vi "Loop Till Force Sensed V2.vi"() -> ()   [LabVIEW 2013]
uses:
  <vilib>/Analysis/baseanly.llb/Mean (DBL).vi
  <vilib>/LabVIEW Interface for Arduino/LabVIEW Interface for Arduino.lvlib
  <vilib>/Analysis/NI_AALBase.lvlib
panel:
  out "Force Threshhold Reached":bool
  out "Force Average":dbl format="%0.2f"
  out "Force vs Time":dbl(graph)
  out "Voltage Average":dbl format="%0.2f"
  in  "Array":dbl[](array[numeric])
  in  "Analog Input Pin":u8
  in  "Stop":bool
  out "Volatege vs Time":dbl(graph)
  out "output array":dbl[](array[numeric])
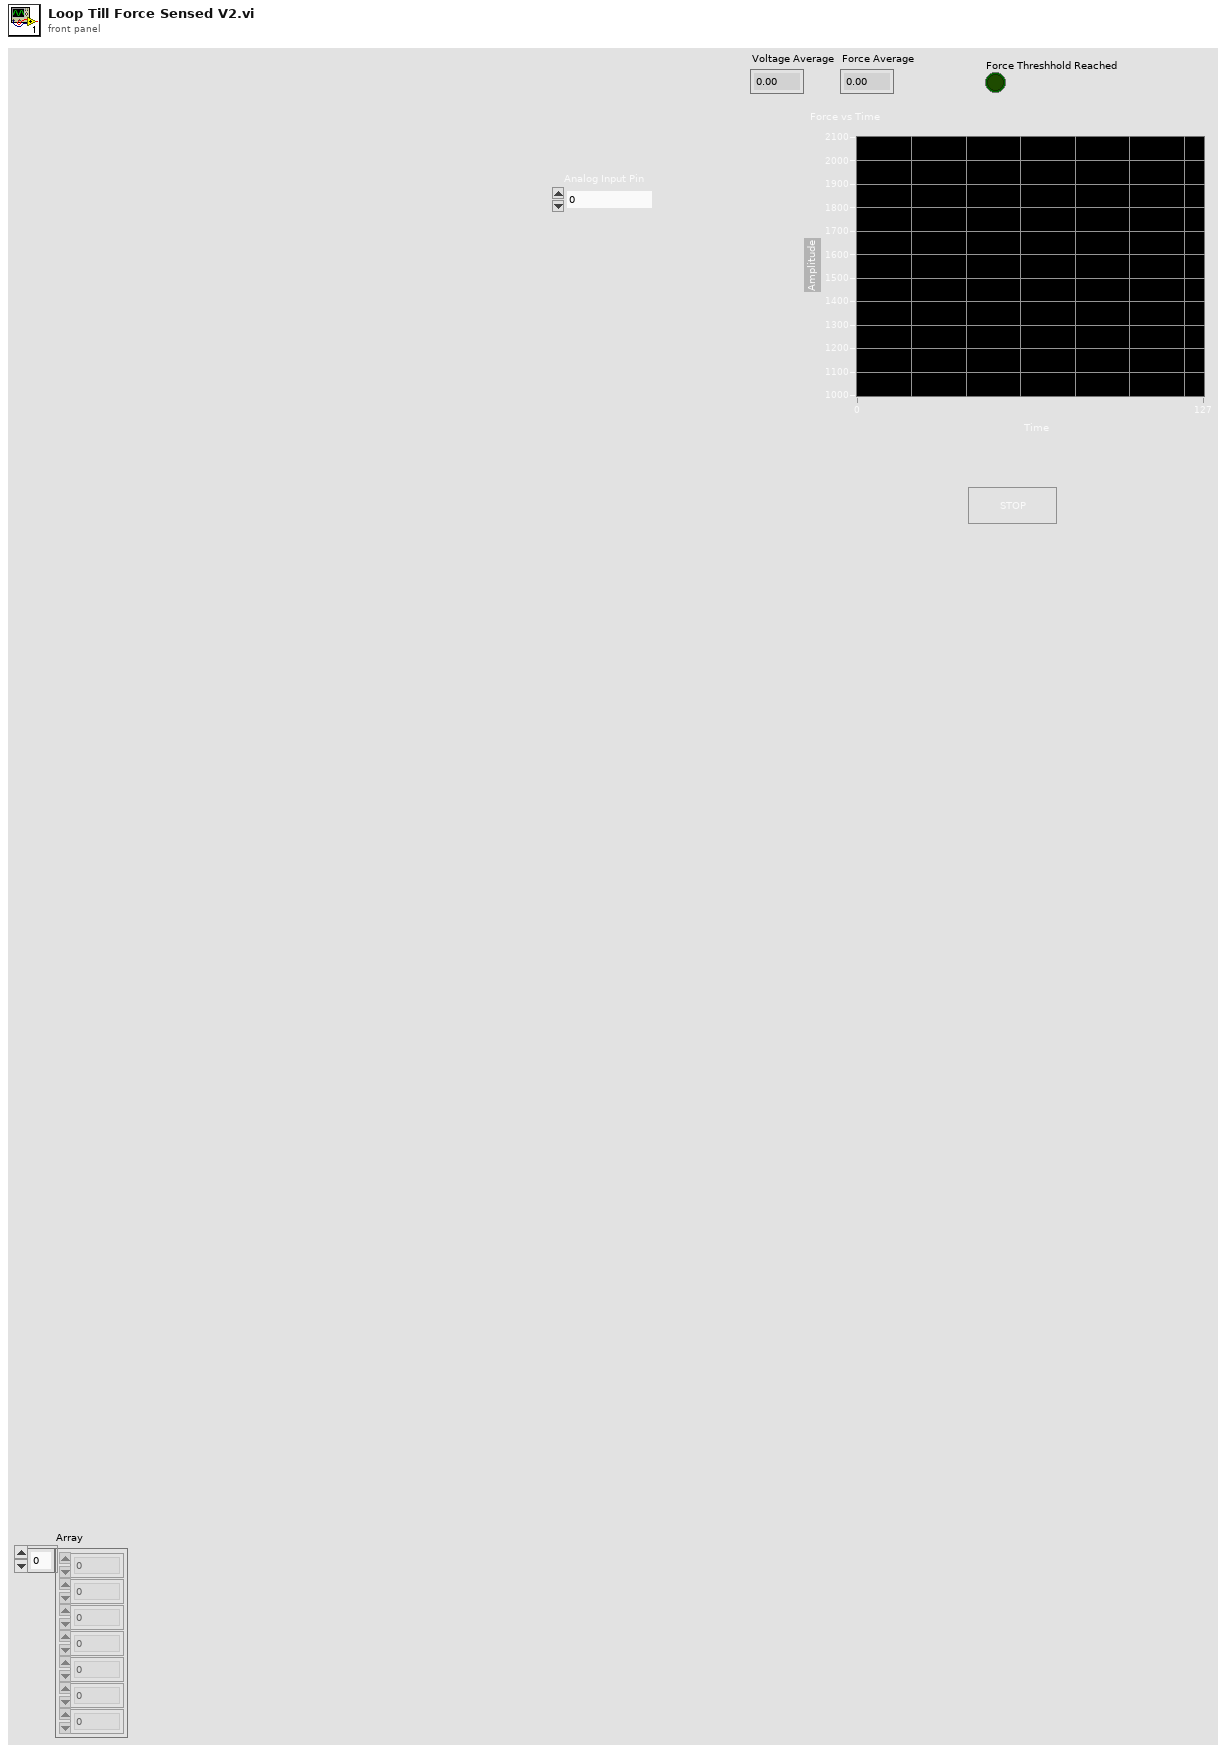
[diagram p1: front panel]
types:
  T1 = typedef "LabVIEW Interface for Arduino.lvlib/Arduino Resource.ctl" = cluster{"VISA resource":refnum<visa-resource-name>, "Board Type":T2, "Connection Type":enum8{"USB / Serial"}, "Bytes Per Packet (15)":u8}
  T2 = typedef "LabVIEW Interface for Arduino.lvlib/Board Type.ctl" = enum16{"Uno", "Dimuelanove w/Atmega 328", "Mega 2560"}
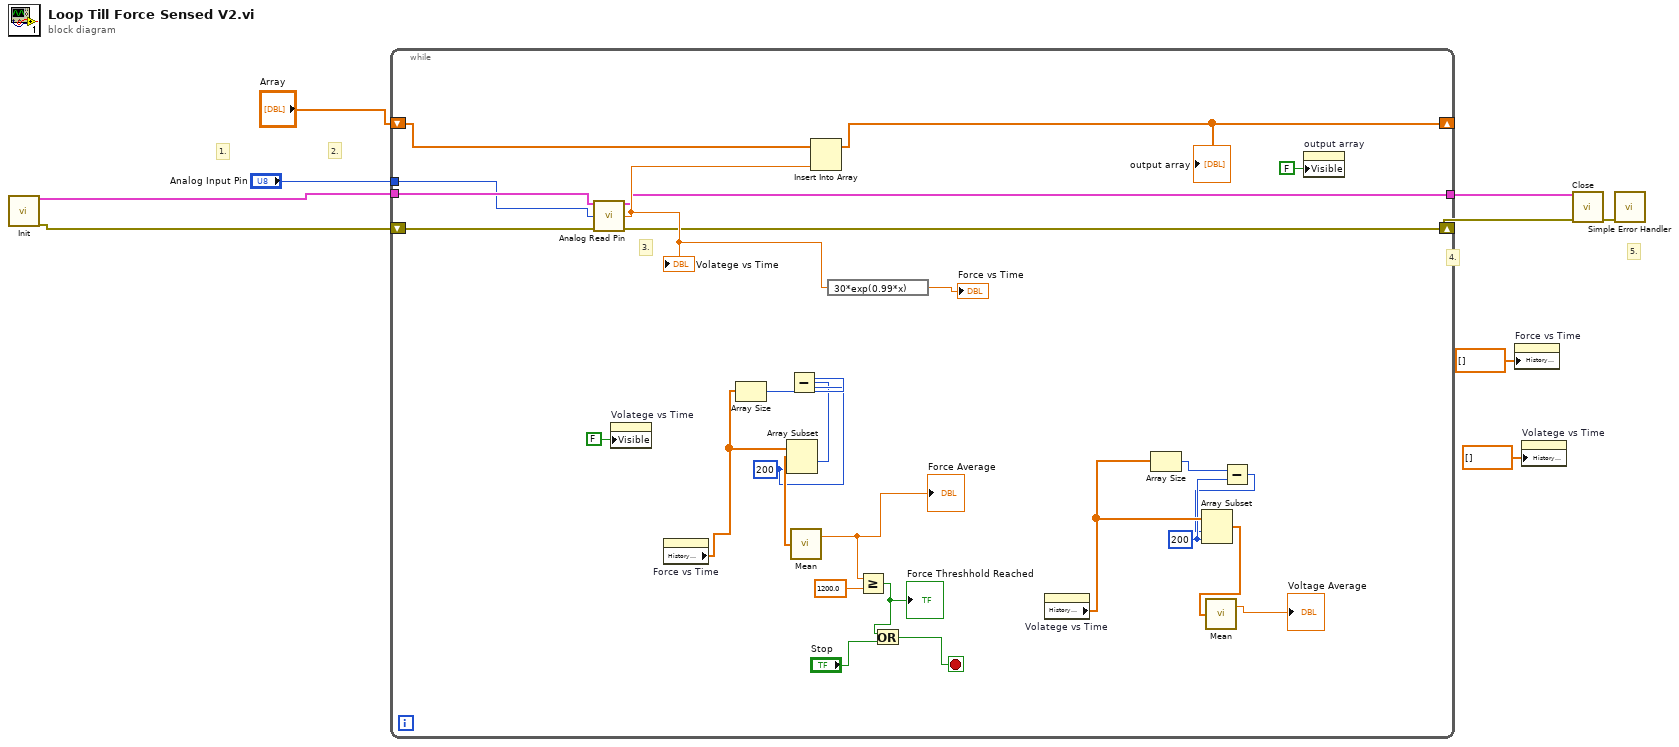
[diagram p0: block diagram]
diagram:
  # "5."
  # "4."
  # "2."
  # "1."
  n1 = call <vilib>:"Init.vi"() -> ("Arduino Resource"=w4:T1, "error out"=w2:errorcluster)  [unwired: 18 in]
  n2 = while {
    shift-right: [w11] -> w8
    shift-left: w2 -> [w12]
    shift-right: [w35] -> _
    shift-left: "Array" -> [w36]
    tunnel: w4 -> [w14]
    tunnel: "Analog Input Pin" -> [w13]
    tunnel: [w10] -> w1
    stop <- w18 stop-if-true
    w27 = 200 ("length")
    w24 = 200 ("length")
    # "3."
    n3 = call <vilib>:"Analog Read Pin.vi"("Arduino Resource"=w14, "Analog Input Pin (0)"=w13, "error in"=w12) -> ("Arduino Resource"=w10:T1, "Voltage"=w15:dbl, "error out"=w11:errorcluster)  [unwired: 10 in]
    "Volatege vs Time" <- w15
    n4 = property on="Volatege vs Time" class="WFChart (strict)"("Visible"=FALSE) -> ()  [unwired: 2 in, 2 out]
    n5 = property on="Force vs Time" class="WFChart (strict)"() -> ("History Data"=w33:dbl[])  [unwired: 2 in, 2 out]
    n6 = Array Size(array=w33) -> (size(s)=w25:i32)
    n7 = Subtract(x=w25, y=w24) -> (x-y=w23:i32)
    n8 = Array Subset(array=w33, index=w23, length=w24) -> (w32:dbl[])
    n9 = call-poly <vilib>:"Mean.vi"("X"=w32) -> ("mean"=w22:dbl)  [unwired: 1 out]
    "Force Average" <- w22
    n10 = Insert Into Array(array=w36, new element=w15) -> (w35:dbl[])  [unwired: 1 in]
    "output array" <- w35
    n11 = expression code="30*exp(0.99*x)"(w15) -> (→"Force vs Time":dbl)
    n12 = Greater Or Equal?(x=w22, y=1200.0) -> (x >= y?=w20:bool)
    "Force Threshhold Reached" <- w20
    n13 = Or(x=w20, y="Stop") -> (x .or. y?=w18:bool)
    n14 = property on="Volatege vs Time" class="WFChart (strict)"() -> ("History Data"=w31:dbl[])  [unwired: 2 in, 2 out]
    n15 = Array Size(array=w31) -> (size(s)=w28:i32)
    n16 = Subtract(x=w28, y=w27) -> (x-y=w26:i32)
    n17 = Array Subset(array=w31, index=w26, length=w27) -> (w29:dbl[])
    n18 = call-poly <vilib>:"Mean.vi"("X"=w29) -> ("mean"=→"Voltage Average":dbl)  [unwired: 1 out]
    n19 = property on="output array" class="Arr (strict)"("Visible"=FALSE) -> ()  [unwired: 2 in, 2 out]
  }
  n20 = property on="Force vs Time" class="WFChart (strict)"("History Data"=dbl[] []) -> ()  [unwired: 2 in, 2 out]
  n21 = property on="Volatege vs Time" class="WFChart (strict)"("History Data"=dbl[] []) -> ()  [unwired: 2 in, 2 out]
  n22 = call <vilib>:"Close.vi"("Arduino Resource"=w1, "error in"=w8) -> ("error out"=w9:errorcluster)  [unwired: 13 in]
  n23 = call <vilib>:"Simple Error Handler.vi"("error in (no error)"=w9) -> ()  [unwired: 4 in, 5 out]
